vi "Color Detector.vi"() -> ()   [LabVIEW 2014]
uses:
  <vilib>/Instr/_visa.llb/VISA Configure Serial Port (Instr).vi
panel:
  out "Voltage":string
  in  "Muestreo":i32
  in  "Stop":bool
  in  "COMM":refnum<visa-resource-name>
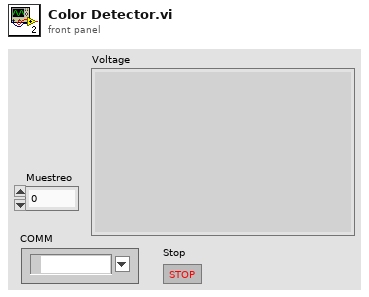
[diagram p1: front panel]
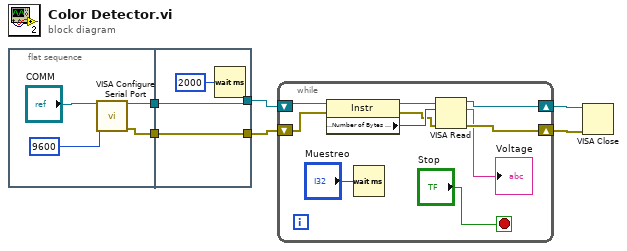
[diagram p0: block diagram]
diagram:
  n1 = flat-sequence {
    tunnel: [w9] -> w6
    tunnel: [w8] -> w4
    tunnel: w6 -> [w12]
    tunnel: [w12] -> w5
    tunnel: [w11] -> w3
    tunnel: w4 -> [w11]
    frame #0 {
      n2 = call-poly "VISA Configure Serial Port"("VISA resource name"="COMM", "baud rate (9600)"=9600) -> ("VISA resource name out"=w8:refnum<visa-resource-name>, "error out"=w9:errorcluster)  [unwired: 12 in]
    }
    frame #1 {
      n3 = Wait (ms)(milliseconds to wait=u32 2000) -> ()  [unwired: 1 out]
    }
  }
  n4 = while {
    shift-right: [w15] -> w1
    shift-left: w5 -> [w20]
    shift-right: [w19] -> w2
    shift-left: w3 -> [w21]
    stop <- "Stop" stop-if-true
    n5 = property class="Instr"(reference=w21, error in=w20) -> (reference out=w18:refnum<visa-resource-name>, error out=w16:errorcluster, "Serial Settings:Number of Bytes at Serial Port"=w17:u32)
    n6 = Wait (ms)(milliseconds to wait="Muestreo") -> ()  [unwired: 1 out]
    n7 = VISA Read(VISA resource name=w18, byte count=w17, error in (no error)=w16) -> (VISA resource name out=w19:refnum<visa-resource-name>, read buffer=→"Voltage":string, error out=w15:errorcluster)  [unwired: 1 out]
  }
  n8 = VISA Close(VISA resource name=w2, error in (no error)=w1) -> ()  [unwired: 1 out]
